vi "Shift_Value_CH1_calibration.vi"(0 "CH1 Val1":dbl, 1 "CH1 Val2":dbl, 2 "CH1 Range IN":dbl, 3 "USB Interface Name":refnum<visa-resource-name>="COM3", 4 "Input buffer size":u32=16384, 5 "error in (no error)":errorcluster, 9 "WRITE":bool, 19 "Sign Value":dbl) -> (6 "MB address":string, 7 "MB value":u8 format="%x", 8 "UB address":string, 10 "HB address":string, 11 "error out":errorcluster, 12 "LB address":string, 13 "UB value":u8 format="%x", 14 "CH1 shift value uV":dbl, 15 "CH1shift val HEX uV":u32 format="%x", 16 "Sign Addrss":string, 17 "HB value":u8 format="%x", 18 "LB value":u8 format="%x")   [LabVIEW 2012]
panel:
  out "LB value":string
  out "HB value":string
  out "UB value":string
  out "MB value":string
  # "1. Computes address based on the input range \"Range IN\"\n2. Take absolute values of positive and negative voltage reads in uV compares them and subtracts smaller value from the larger one. The result is devided by 2.\nIf VAL1>VAL2: ( |VAL1| - |VAL2| )/ 2"
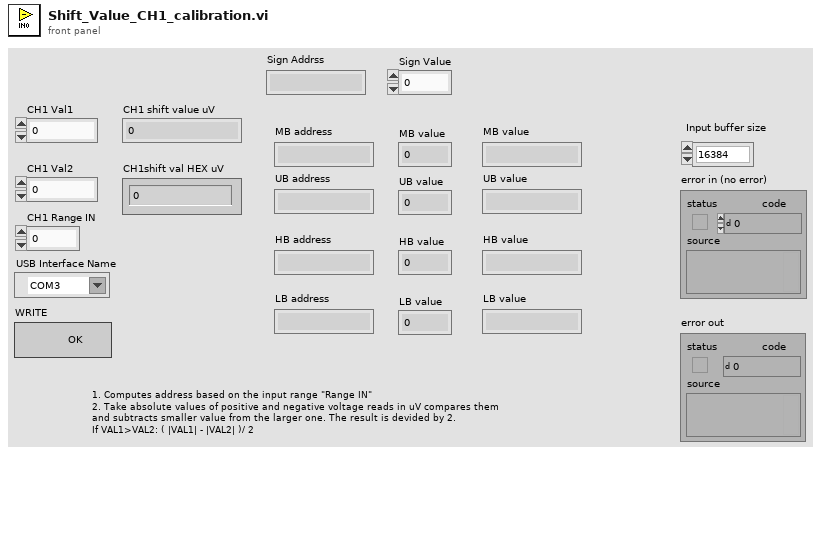
[diagram p1: front panel]
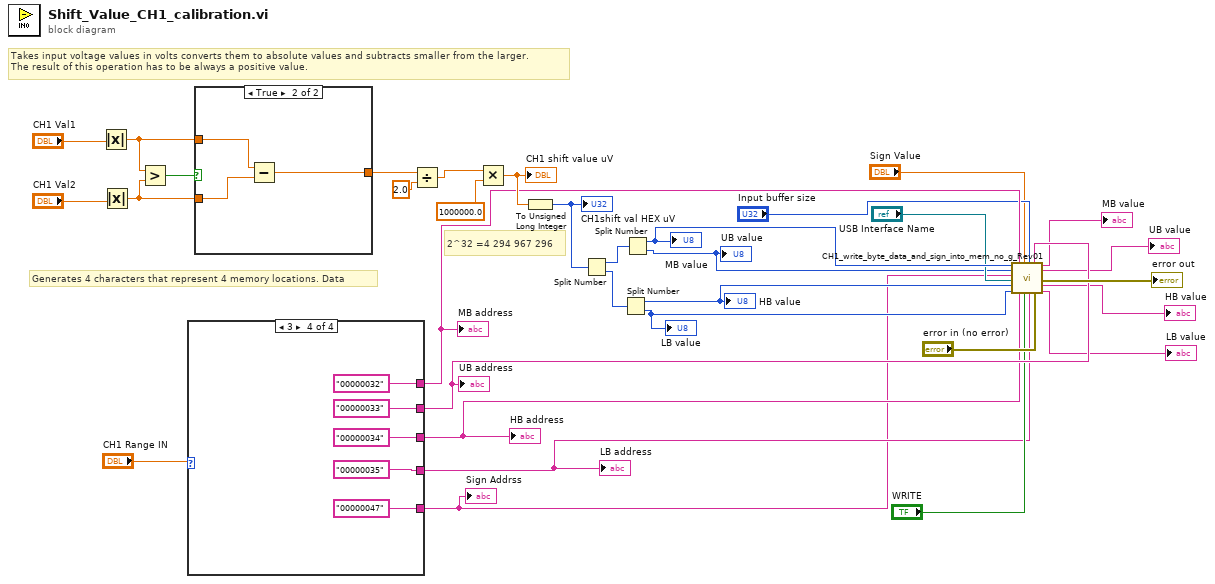
[diagram p0: block diagram]
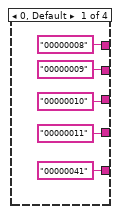
[diagram p2: hidden frame]
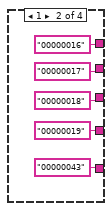
[diagram p3: hidden frame]
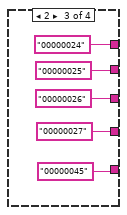
[diagram p4: hidden frame]
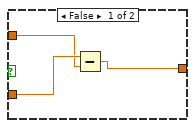
[diagram p5: hidden frame]
diagram:
  # "2^32 =4 294 967 296"
  # "Generates 4 characters that represent 4 memory locations. Data"
  # "Takes input voltage values in volts converts them to absolute values and subtracts smaller from the larger.\nThe result of this operation has to be always a positive value."
  n1 = Absolute Value(x="CH1 Val1") -> (abs(x)=w30:dbl)
  n2 = Absolute Value(x="CH1 Val2") -> (abs(x)=w29:dbl)
  n3 = Greater?(x=w30, y=w29) -> (0:w31:bool)
  n4 = case shown="3" "CH1 Range IN" {
    tunnel: ["00000008" "00000016" "00000024" "00000032"] -> w12
    tunnel: ["00000009" "00000017" "00000025" "00000033"] -> w11
    tunnel: ["00000010" "00000018" "00000026" "00000034"] -> w10
    tunnel: ["00000011" "00000019" "00000027" "00000035"] -> w8
    tunnel: ["00000041" "00000043" "00000045" "00000047"] -> w1
    frame 0, Default {
    }
    frame 1 {
    }
    frame 2 {
    }
    frame 3 {
    }
  }
  "MB address" <- w12
  "UB address" <- w11
  "HB address" <- w10
  "LB address" <- w8
  "Sign Addrss" <- w1
  n5 = case shown="True" w31 {
    tunnel: w30 -> [w55 w59]
    tunnel: w29 -> [w56 w58]
    tunnel: [w54 w57] -> w28
    frame False {
      n6 = Subtract(x=w56, y=w55) -> (x-y=w54:dbl)
    }
    frame True {
      n7 = Subtract(x=w59, y=w58) -> (x-y=w57:dbl)
    }
  }
  n8 = Divide(x=w28, y=2.0) -> (x/y=w26:dbl)
  n9 = Multiply(x=w26, y=1000000.0) -> (x*y=w24:dbl)
  "CH1 shift value uV" <- w24
  n10 = To Unsigned Long Integer(number=w24) -> (unsigned 32bit integer=w23:u32)
  "CH1shift val HEX uV" <- w23
  n11 = Split Number(x=w23) -> (hi(x)=w22:u16, lo(x)=w21:u16)
  n12 = Split Number(x=w21) -> (hi(x)=w14:u8, lo(x)=w13:u8)
  "HB value" <- w14
  "LB value" <- w13
  n13 = Split Number(x=w22) -> (hi(x)=w19:u8, lo(x)=w15:u8)
  "MB value" <- w19
  "UB value" <- w15
  n14 = call "CH1_write_byte_data_and_sign_into_mem_no_g_Rev01.vi"("MB data"=w19, "UB data"=w15, "Address of the sign"=w1, "USB Interface Name"="USB Interface Name", "HB data"=w14, "LB data"=w13, "MB address"=w12, "HB address"=w10, "Sign Value"="Sign Value", "WRITE DATA"="WRITE", "Input buffer size"="Input buffer size", "LB address"=w8, "UB address"=w11, "error in (no error)"="error in (no error)") -> ("MB data string"=→"MB value":string, "UB data string"=→"UB value":string, "error out"=→"error out":errorcluster, "HB data string"=→"HB value":string, "LB data string"=→"LB value":string)  [unwired: 1 in]
